vi "day 7 task 2.vi"() -> ()   [LabVIEW 2019]
panel:
  out "deleteme":u64
  out "sum pt 1":u64
  out "element":map{string, u64}(c390)
  out "String":string
  out "map":T1(c390)
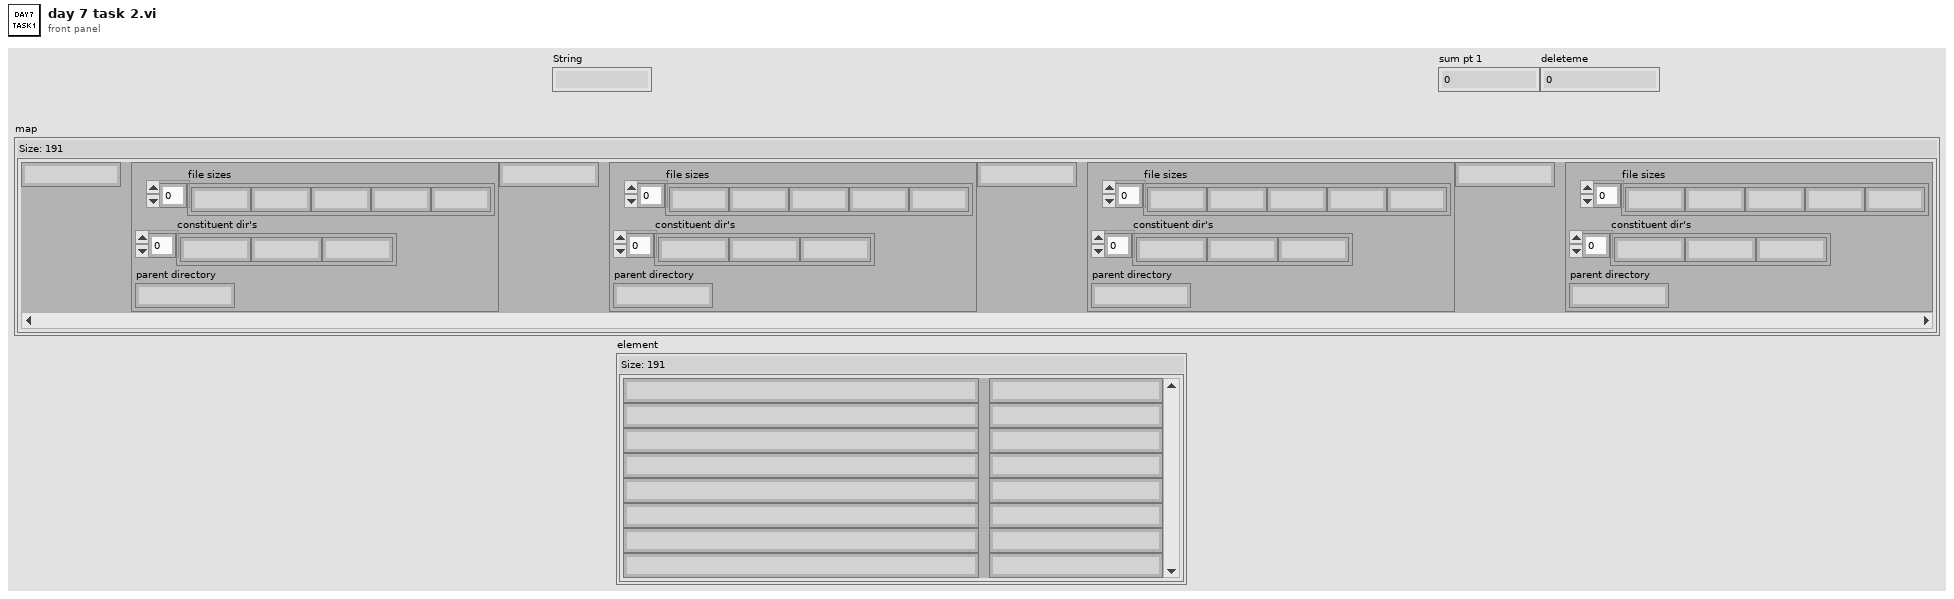
[diagram p1: front panel]
types:
  T1 = map{string, cluster{"file sizes":u64[], "constituent dir's":string[], "parent directory":string}}
  T2 = cluster{"file sizes":u64[], "constituent dir's":string[], "parent directory":string}
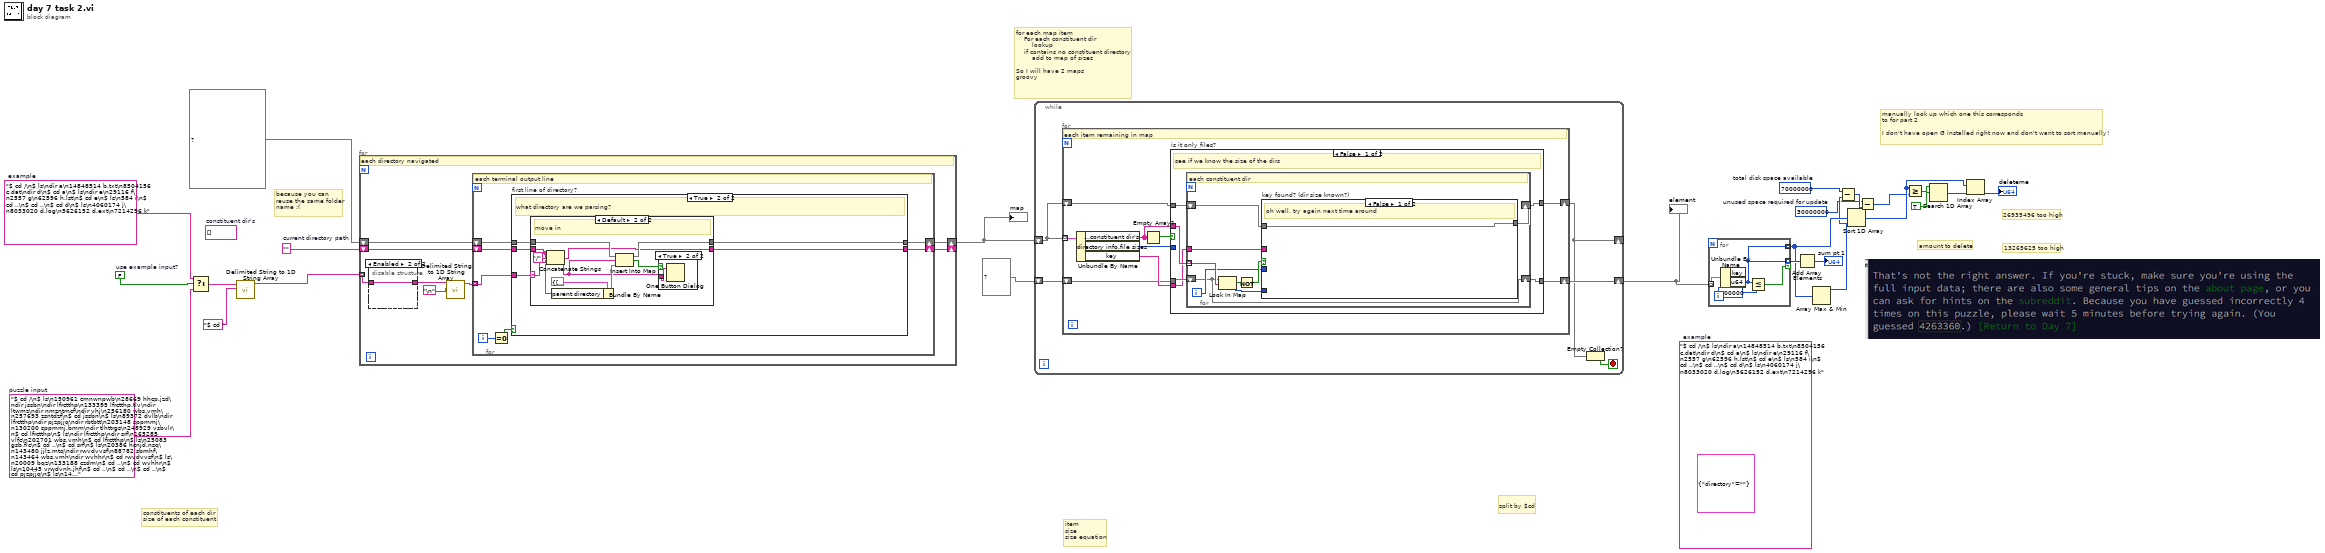
[diagram p0: block diagram]
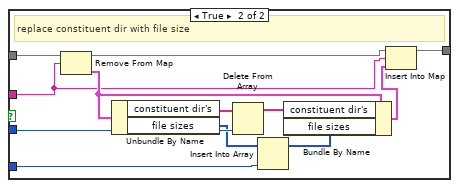
[diagram p2: hidden frame]
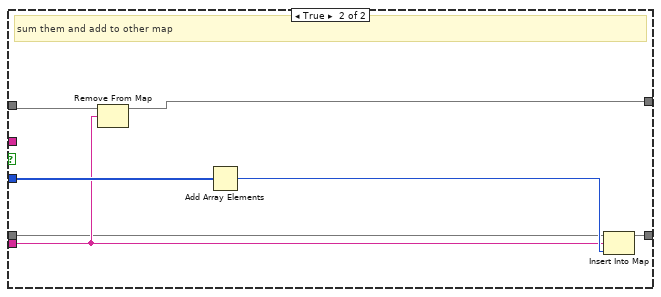
[diagram p3: hidden frame]
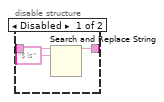
[diagram p4: hidden frame]
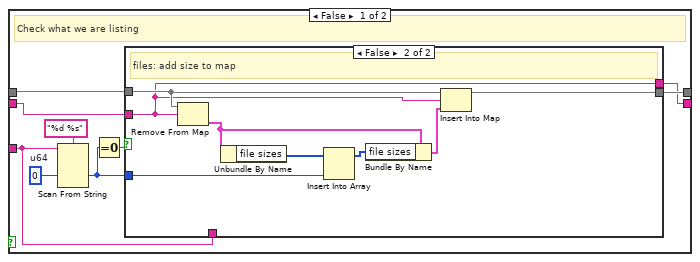
[diagram p5: hidden frame]
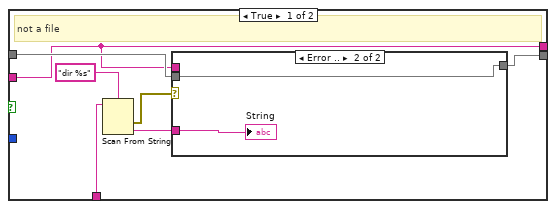
[diagram p6: hidden frame]
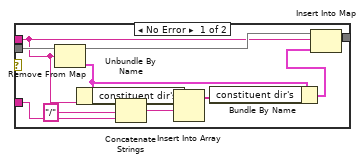
[diagram p7: hidden frame]
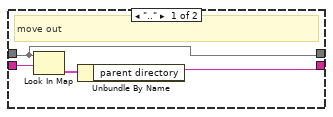
[diagram p8: hidden frame]
diagram:
  w1 = u64 30000000  # unused space required for update
  w12 = u64 70000000  # total disk space available
  w17 = ""  # current directory path
  (unwired) string[] []  # constituent dir's
  (unwired) cluster{"directory":string} {"directory"=""}
  (unwired) "$ cd /\n$ ls\ndir a\n14848514 b.txt\n8504156 c.dat\ndir d\n$ cd a\n$ ls\ndir e\n29116 f\n2557 g\n62596 h.lst\n$ cd e\n$ ls\n584 i\n$ cd ..\n$ cd ..\n$ cd d\n$ ls\n4060174 j\n8033020 d.log\n5626152 d.ext\n7214296 k"  # example
  w22 = "$ cd /\n$ ls\ndir a\n14848514 b.txt\n8504156 c.dat\ndir d\n$ cd a\n$ ls\ndir e\n29116 f\n2557 g\n62596 h.lst\n$ cd e\n$ ls\n584 i\n$ cd ..\n$ cd ..\n$ cd d\n$ ls\n4060174 j\n8033020 d.log\n5626152 d.ext\n7214296 k"  # example
  w23 = FALSE  # use example input?
  w24 = "$ cd /\n$ ls\n150961 cmnwnpwb\n28669 hhcp.jzd\ndir jssbn\ndir lfrctthp\n133395 lfrctthp.tlv\ndir ltwmz\ndir nmzntmcf\ndir vhj\n256180 wbs.vmh\n257693 zsntdzf\n$ cd jssbn\n$ ls\n89372 dvlb\ndir lfrctthp\ndir pjzpjjq\ndir rbtbtt\n203148 sppmmj\n130200 sppmmj.bmm\ndir tlhttrgs\n248929 vsbvlr\n$ cd lfrctthp\n$ ls\ndir lfrctthp\ndir srf\n165285 vlfc\n202701 wbs.vmh\n$ cd lfrctthp\n$ ls\n25083 gsb.flc\n$ cd ..\n$ cd srf\n$ ls\n20386 hcnjd.nsq\n143480 jjlz.mtq\ndir rwvdvvsf\n88782 sbmhf\n143464 wbs.vmh\ndir wvhhr\n$ cd rwvdvvsf\n$ ls\n20009 bqz\n133188 czdm\n$ cd ..\n$ cd wvhhr\n$ ls\n10445 vrwdvnh.jhf\n$ cd ..\n$ cd ..\n$ cd ..\n$ cd pjzpjjq\n$ ls\n14329 chgbd.zjf\ndir dvlb\n212284 pjc\ndir qlrn\n225566 rhzgmnb.nhd\n145766 sppmmj.dzz\ndir vpltwcs\n125853 wbs.vmh\n$ cd dvlb\n$ ls\ndir bjfqsb\ndir fnwsmj\n154127 gplzm\n264923 qcp.qvc\ndir wlhfvwl\ndir wrgqqts\ndir zhj\n$ cd bjfqsb\n$ ls\ndir jgltcw\n$ cd jgltcw\n$ ls\n264579 shmqqjf.fwd\n$ cd ..\n$ cd ..\n$ cd fnwsmj\n$ ls\ndir lfrctthp\ndir rddpmj\n$ cd lfrctthp\n$ ls\ndir qdgqdtn\n198919 qhjbh.fbc\ndir sgddcfdn\n$ cd qdgqdtn\n$ ls\n230357 lbcgfp.vzq\n$ cd ..\n$ cd sgddcfdn\n$ ls\n110212 cwjbzd.npb\ndir lnjln\n207550 wlvdsjj\n$ cd lnjln\n$ ls\n28970 tdw\n$ cd ..\n$ cd ..\n$ cd ..\n$ cd rddpmj\n$ ls\ndir fhlnmw\n$ cd fhlnmw\n$ ls\n228871 mcgdrzg\n$ cd ..\n$ cd ..\n$ cd ..\n$ cd wlhfvwl\n$ ls\ndir rbwq\n$ cd rbwq\n$ ls\n139444 jdczdlwb\n66039 mnbq.sdq\n$ cd ..\n$ cd ..\n$ cd wrgqqts\n$ ls\n124869 dvlb.cfl\n$ cd ..\n$ cd zhj\n$ ls\ndir hww\n192363 lqn\ndir nqv\n$ cd hww\n$ ls\n14681 czhd.bdn\n232222 fgcfbrs.wqt\ndir pnsbrd\n155416 vsw.npv\n199792 wbs.vmh\n44877 znpdrr.rmd\n$ cd pnsbrd\n$ ls\n179442 vsbvlr\n55431 zbhj.wnh\n$ cd ..\n$ cd ..\n$ cd nqv\n$ ls\n262693 hnz.czd\n259429 lptljbz\ndir rjgbm\ndir tlhttrgs\n76496 tlhttrgs.jlv\n260003 vsbvlr\n$ cd rjgbm\n$ ls\n45885 fgfh.tch\n42899 lfrctthp.fbc\n159401 nnmg.tvz\n144595 trzgtn.scg\n$ cd ..\n$ cd tlhttrgs\n$ ls\ndir cqtnvzn\n220458 wbs.vmh\n$ cd cqtnvzn\n$ ls\n49609 czdm\n$ cd ..\n$ cd ..\n$ cd ..\n$ cd ..\n$ cd ..\n$ cd qlrn\n$ ls\n150270 bflnzt\n203988 bgq\ndir jwgd\n256702 sppmmj\ndir wbgvqpc\n$ cd jwgd\n$ ls\n57414 lmlbtpg.wdp\n$ cd ..\n$ cd wbgvqpc\n$ ls\ndir dvlb\ndir qfhvjtv\ndir tpcwhmv\n$ cd dvlb\n$ ls\n118388 hhcp.jzd\n$ cd ..\n$ cd qfhvjtv\n$ ls\n82966 lfrctthp\ndir mhbbpdpj\n139234 wbs.vmh\n$ cd mhbbpdpj\n$ ls\ndir ghrbbh\n$ cd ghrbbh\n$ ls\n24686 tlhttrgs\n$ cd ..\n$ cd ..\n$ cd ..\n$ cd tpcwhmv\n$ ls\n3666 hhcp.jzd\n$ cd ..\n$ cd ..\n$ cd ..\n$ cd vpltwcs\n$ ls\ndir tlhttrgs\n146745 vsbvlr\n$ cd tlhttrgs\n$ ls\ndir cchd\n32682 cvbr.rmh\n209102 mpdpnb\n96179 wbs.vmh\n$ cd cchd\n$ ls\n126044 wmrv\n$ cd ..\n$ cd ..\n$ cd ..\n$ cd ..\n$ cd rbtbtt\n$ ls\n169793 hzgdsb.tbs\ndir wqmvzg\n$ cd wqmvzg\n$ ls\ndir lzbj\n$ cd lzbj\n$ ls\ndir tnhdmqjh\n$ cd tnhdmqjh\n$ ls\n5150 lfrctthp\n$ cd ..\n$ cd ..\n$ cd ..\n$ cd ..\n$ cd tlhttrgs\n$ ls\ndir zjghthcb\ndir zmlpwlm\n$ cd zjghthcb\n$ ls\ndir dvlb\ndir ghzsqrn\ndir hvwjc\ndir lfrctthp\n$ cd dvlb\n$ ls\n167639 dvlb.fhs\n70305 qnhgn.mgn\n$ cd ..\n$ cd ghzsqrn\n$ ls\n74556 dbrtz.lrn\ndir fngzpjm\ndir mdqbvhrr\n220711 mrfjpgwj\ndir sfhqmzhd\n67424 tlhttrgs.thf\n202325 vsngvn.ttq\n$ cd fngzpjm\n$ ls\ndir dvlb\ndir ghzwdw\n$ cd dvlb\n$ ls\n59824 bmvzg\n184952 lfrctthp\n51434 qwcttnh.pbs\n206348 wbs.vmh\n$ cd ..\n$ cd ghzwdw\n$ ls\n132594 lfrctthp\n99032 tlhttrgs.cvp\n$ cd ..\n$ cd ..\n$ cd mdqbvhrr\n$ ls\n32598 zsfv.qqv\n$ cd ..\n$ cd sfhqmzhd\n$ ls\n58893 wpmbm\n$ cd ..\n$ cd ..\n$ cd hvwjc\n$ ls\n233454 ccpnsjm.cwc\n72232 lfrctthp\ndir nchvqtdq\n248368 ptrlpt.gdf\n222059 qgjv\n69105 wbs.vmh\ndir wnj\n$ cd nchvqtdq\n$ ls\n49931 gjwjq.jrc\n$ cd ..\n$ cd wnj\n$ ls\n182139 ccpnsjm.cwc\ndir dvlb\n72806 hhcp.jzd\n156378 sppmmj\n$ cd dvlb\n$ ls\ndir cwjbzd\n$ cd cwjbzd\n$ ls\ndir tlhttrgs\n$ cd tlhttrgs\n$ ls\n240264 vdp.wzt\n$ cd ..\n$ cd ..\n$ cd ..\n$ cd ..\n$ cd ..\n$ cd lfrctthp\n$ ls\n168164 ccpnsjm.cwc\n68428 dcmfjn\n133121 dvlb\n146217 sppmmj.zjm\ndir thgh\ndir zzffz\n$ cd thgh\n$ ls\ndir nrntbh\ndir qlhbf\n$ cd nrntbh\n$ ls\n139964 lfrctthp.brp\n$ cd ..\n$ cd qlhbf\n$ ls\n115891 vsbvlr\n$ cd ..\n$ cd ..\n$ cd zzffz\n$ ls\n170513 tlhttrgs.hsw\n$ cd ..\n$ cd ..\n$ cd ..\n$ cd zmlpwlm\n$ ls\n232644 wvjrtvps.hrb\n$ cd ..\n$ cd ..\n$ cd ..\n$ cd lfrctthp\n$ ls\ndir cwjbzd\ndir dvlb\n65658 fclf\n191985 hhcp.jzd\ndir lwqdqm\ndir mpb\ndir ndn\ndir rtpwjds\n185299 smp\ndir sqhvvsb\ndir vzh\ndir zzvnq\n$ cd cwjbzd\n$ ls\n172122 ccpnsjm.cwc\ndir dfqpqqw\ndir lfrctthp\n123102 lfrctthp.cms\n73991 lqhjcbms\n207693 mcnwp\ndir sppmmj\n114128 tzrrgl\n$ cd dfqpqqw\n$ ls\n67239 dgssm.crl\ndir rjm\n$ cd rjm\n$ ls\n25830 nnwdzf\n$ cd ..\n$ cd ..\n$ cd lfrctthp\n$ ls\ndir fqswn\n241343 jllwj.wjc\n$ cd fqswn\n$ ls\n76154 ccpnsjm.cwc\ndir dhgghnm\ndir vpbwj\n$ cd dhgghnm\n$ ls\n36757 jbmlssv.ndp\ndir sppmmj\n$ cd sppmmj\n$ ls\ndir dsss\n$ cd dsss\n$ ls\n201519 vsbvlr\n$ cd ..\n$ cd ..\n$ cd ..\n$ cd vpbwj\n$ ls\n154042 ccpnsjm.cwc\ndir tlhttrgs\n271666 vsbvlr\n$ cd tlhttrgs\n$ ls\n125785 cwjbzd.lqr\n19315 jdcm.mrz\n$ cd ..\n$ cd ..\n$ cd ..\n$ cd ..\n$ cd sppmmj\n$ ls\ndir sppmmj\n$ cd sppmmj\n$ ls\n161387 fwh.wtt\n$ cd ..\n$ cd ..\n$ cd ..\n$ cd dvlb\n$ ls\ndir dnqvhtr\ndir jqpzj\ndir jvvsgbl\ndir tlhttrgs\n$ cd dnqvhtr\n$ ls\ndir jzm\ndir phcfgqfs\ndir sppmmj\ndir vhrst\n$ cd jzm\n$ ls\n143413 sgsbj.qtr\ndir smtpdcpf\n$ cd smtpdcpf\n$ ls\n95947 lgzlj\n$ cd ..\n$ cd ..\n$ cd phcfgqfs\n$ ls\n257801 hhcp.jzd\n$ cd ..\n$ cd sppmmj\n$ ls\n230280 ccpnsjm.cwc\n261954 hhcp.jzd\ndir hmcn\ndir mrhsrrm\ndir nlqmghj\ndir rqbtcvfw\n70788 vsbvlr\n114344 wbs.vmh\n225265 wjnf.wrv\n$ cd hmcn\n$ ls\n206476 dvlb\n214973 lfrctthp\n$ cd ..\n$ cd mrhsrrm\n$ ls\n126589 wbs.vmh\n$ cd ..\n$ cd nlqmghj\n$ ls\n113621 mdqvh.flp\n$ cd ..\n$ cd rqbtcvfw\n$ ls\n259673 wbs.vmh\n$ cd ..\n$ cd ..\n$ cd vhrst\n$ ls\n102273 sppmmj\n$ cd ..\n$ cd ..\n$ cd jqpzj\n$ ls\n7675 vwls.wjz\n$ cd ..\n$ cd jvvsgbl\n$ ls\n217539 bgjgtfbv.wcf\ndir fbvls\ndir gtwrhhd\ndir tlhttrgs\n59720 wbs.vmh\n$ cd fbvls\n$ ls\n146823 ccpnsjm.cwc\n$ cd ..\n$ cd gtwrhhd\n$ ls\n59762 wbs.vmh\n$ cd ..\n$ cd tlhttrgs\n$ ls\n7093 ccpnsjm.cwc\ndir dvlb\ndir hjclnb\n$ cd dvlb\n$ ls\n62683 trww\n$ cd ..\n$ cd hjclnb\n$ ls\n245444 bcnlmstj.bsj\n167166 czdm\n$ cd ..\n$ cd ..\n$ cd ..\n$ cd tlhttrgs\n$ ls\n53060 czdm\n217177 hzwn\n$ cd ..\n$ cd ..\n$ cd lwqdqm\n$ ls\ndir bdgnmf\ndir dvlb\n89596 vsbvlr\n$ cd bdgnmf\n$ ls\n146880 wbs.vmh\n$ cd ..\n$ cd dvlb\n$ ls\n184438 vsbvlr\n$ cd ..\n$ cd ..\n$ cd mpb\n$ ls\ndir dvlb\n$ cd dvlb\n$ ls\ndir prqfqf\n$ cd prqfqf\n$ ls\ndir ltmjppj\n$ cd ltmjppj\n$ ls\n241963 bjgzsq.srr\n$ cd ..\n$ cd ..\n$ cd ..\n$ cd ..\n$ cd ndn\n$ ls\n184702 cnv.vtn\n52486 dvlb\ndir hfq\n52100 hswnvlq.frd\n$ cd hfq\n$ ls\ndir bsjgglbs\n263904 cwjbzd.sht\n265639 phpvlfw.jmm\n178105 wbs.vmh\n25124 wcq.qct\n$ cd bsjgglbs\n$ ls\n121761 czdm\n$ cd ..\n$ cd ..\n$ cd ..\n$ cd rtpwjds\n$ ls\n117111 qjvrwsfl\n132235 rwjf\ndir sdssvrst\n223399 wjfdgt.ldj\n$ cd sdssvrst\n$ ls\n114380 ccpnsjm.cwc\n$ cd ..\n$ cd ..\n$ cd sqhvvsb\n$ ls\n7812 gjhj\n239114 hhcp.jzd\ndir ldmwm\n230777 vsbvlr\n$ cd ldmwm\n$ ls\n67855 blcbqb.wpz\ndir cwjbzd\n250365 czdm\n249613 dvlb.mfq\ndir jdsbt\n95934 tlhttrgs.wgw\n$ cd cwjbzd\n$ ls\n147822 cwjbzd.lff\n122632 hhcp.jzd\ndir llcflrds\ndir tlhttrgs\n67326 tvptb.fzl\ndir wtcttdzg\n$ cd llcflrds\n$ ls\ndir cngdgq\n$ cd cngdgq\n$ ls\n235724 lqqcfphg\n$ cd ..\n$ cd ..\n$ cd tlhttrgs\n$ ls\ndir cgf\n67714 csb.hcw\ndir cwjbzd\ndir jvs\n119180 lfrctthp.qgm\ndir ppsmqwn\ndir qqmtj\ndir qzmpwzvz\ndir zmsbqrqf\n$ cd cgf\n$ ls\ndir dvlb\n$ cd dvlb\n$ ls\n77864 thff\n$ cd ..\n$ cd ..\n$ cd cwjbzd\n$ ls\n208459 ccpnsjm.cwc\n17127 dtqglmf.zgb\n$ cd ..\n$ cd jvs\n$ ls\n142337 cwjbzd\n$ cd ..\n$ cd ppsmqwn\n$ ls\n147277 rmwh\n$ cd ..\n$ cd qqmtj\n$ ls\n153442 vqld.lsd\n$ cd ..\n$ cd qzmpwzvz\n$ ls\n223666 cwjbzd.gjl\n254370 gjc\n$ cd ..\n$ cd zmsbqrqf\n$ ls\n193665 tjwclf.nzs\n$ cd ..\n$ cd ..\n$ cd wtcttdzg\n$ ls\n52882 hhcp.jzd\n110104 hqwgl.mtb\n$ cd ..\n$ cd ..\n$ cd jdsbt\n$ ls\n77115 ccpnsjm.cwc\n242705 dvlb\n12624 lfrctthp\n145552 sppmmj\n198997 vsbvlr\n$ cd ..\n$ cd ..\n$ cd ..\n$ cd vzh\n$ ls\ndir ccbjg\n91733 czdm\n89195 dvlb\n212167 rvfpbl.rtq\n224909 tlhttrgs.djt\n72916 vpznzhs.dcd\n$ cd ccbjg\n$ ls\ndir mcvsbd\ndir sppmmj\n$ cd mcvsbd\n$ ls\ndir cwjbzd\ndir rbsv\n$ cd cwjbzd\n$ ls\n224826 ccpnsjm.cwc\n$ cd ..\n$ cd rbsv\n$ ls\n164816 lfrctthp\n$ cd ..\n$ cd ..\n$ cd sppmmj\n$ ls\n85264 ccpnsjm.cwc\n104511 dvlb.qgj\n183533 lfrctthp.zdn\n98525 wbs.vmh\n$ cd ..\n$ cd ..\n$ cd ..\n$ cd zzvnq\n$ ls\n107390 lfrctthp\ndir lznpqbrd\ndir pddfg\n143496 prnjh.sgb\ndir pvdz\ndir vnmhs\n118674 zhnh.mpl\n$ cd lznpqbrd\n$ ls\n157950 dpvcgj.wlw\ndir dvlb\n175412 dvlb.qvr\ndir lfrctthp\n84587 pmsjdj\n$ cd dvlb\n$ ls\n41223 rwr.nbz\n$ cd ..\n$ cd lfrctthp\n$ ls\n26056 fqc.fnl\n28191 lgjlw.vql\ndir sppmmj\n262066 wbs.vmh\n$ cd sppmmj\n$ ls\n246742 ccpnsjm.cwc\n$ cd ..\n$ cd ..\n$ cd ..\n$ cd pddfg\n$ ls\ndir cwjbzd\ndir jbw\n147410 vsbvlr\n$ cd cwjbzd\n$ ls\n197956 jpzb.dcw\n$ cd ..\n$ cd jbw\n$ ls\n247206 vsbvlr\n$ cd ..\n$ cd ..\n$ cd pvdz\n$ ls\ndir jctpqbgw\n153177 qwcgjttm.lzm\n94686 vsbvlr\n$ cd jctpqbgw\n$ ls\n190424 qvm\n$ cd ..\n$ cd ..\n$ cd vnmhs\n$ ls\n16118 sdhmzhlg.blf\n$ cd ..\n$ cd ..\n$ cd ..\n$ cd ltwmz\n$ ls\n243152 bdmz\n$ cd ..\n$ cd nmzntmcf\n$ ls\ndir jqcms\ndir lrtsts\ndir lvchpdf\ndir qpzqp\ndir qrgh\ndir scwnmrds\n$ cd jqcms\n$ ls\n105562 ccpnsjm.cwc\n257512 chpr.zvl\ndir cwjbzd\ndir jzqbnpn\ndir ssr\n117496 tlhttrgs.thg\n72550 vsbvlr\n$ cd cwjbzd\n$ ls\ndir mwvlhzdn\ndir qrpllg\n205638 sppmmj.gcz\n$ cd mwvlhzdn\n$ ls\n272658 dvlb.bbw\n$ cd ..\n$ cd qrpllg\n$ ls\n215810 wbs.vmh\n$ cd ..\n$ cd ..\n$ cd jzqbnpn\n$ ls\n112583 sppmmj\n$ cd ..\n$ cd ssr\n$ ls\n66781 hpfpw.pvn\n138840 zhwplzd.wrq\n$ cd ..\n$ cd ..\n$ cd lrtsts\n$ ls\ndir drtrdnsg\n41195 dvlb.fgt\ndir lfrctthp\n$ cd drtrdnsg\n$ ls\ndir gnc\ndir sppmmj\n$ cd gnc\n$ ls\n127922 ccpnsjm.cwc\n233097 lfrctthp\n24075 qtglzq\n$ cd ..\n$ cd sppmmj\n$ ls\n128955 czdm\n64809 jtjh.nzq\ndir mdmh\ndir nbzh\n126095 wbs.vmh\ndir wwhbgg\n$ cd mdmh\n$ ls\ndir zvtjfz\n$ cd zvtjfz\n$ ls\n142470 ptp.qbf\n$ cd ..\n$ cd ..\n$ cd nbzh\n$ ls\n7112 ccpnsjm.cwc\n215395 chrtbjf.fwr\n145865 wld.pdl\n$ cd ..\n$ cd wwhbgg\n$ ls\n51752 hhcp.jzd\n$ cd ..\n$ cd ..\n$ cd ..\n$ cd lfrctthp\n$ ls\n198780 hhcp.jzd\n$ cd ..\n$ cd ..\n$ cd lvchpdf\n$ ls\n108580 hhcp.jzd\n105301 jpjjhshl\ndir njfmmj\ndir nsw\ndir sppmmj\ndir tlhttrgs\ndir tvsvr\n$ cd njfmmj\n$ ls\ndir bjsvdfrf\ndir gjgftj\ndir sppmmj\n25879 twzprtcf.hgl\n$ cd bjsvdfrf\n$ ls\n77668 vsbvlr\n$ cd ..\n$ cd gjgftj\n$ ls\ndir mjbw\n56593 vsbvlr\n$ cd mjbw\n$ ls\n243595 ccpnsjm.cwc\n$ cd ..\n$ cd ..\n$ cd sppmmj\n$ ls\ndir qzvwhr\n$ cd qzvwhr\n$ ls\ndir cwjbzd\n$ cd cwjbzd\n$ ls\n262825 wbs.vmh\n$ cd ..\n$ cd ..\n$ cd ..\n$ cd ..\n$ cd nsw\n$ ls\n210254 rgqpq\n$ cd ..\n$ cd sppmmj\n$ ls\n55463 cwjbzd.dtt\n196779 dvlb\n125377 hgb.qmj\ndir rdd\ndir tlhttrgs\n222280 tspz\ndir zbq\n$ cd rdd\n$ ls\n20045 srmsmr\n$ cd ..\n$ cd tlhttrgs\n$ ls\n47256 wbs.vmh\n$ cd ..\n$ cd zbq\n$ ls\n223951 cwjbzd.vrm\n$ cd ..\n$ cd ..\n$ cd tlhttrgs\n$ ls\n56808 jvndrcmd.ftl\ndir mjcmhg\n220385 prh.wtz\n231575 pzbtlg.fzv\n11100 sqfr.lzs\ndir tlhttrgs\n$ cd mjcmhg\n$ ls\n214188 llsfnv.dmc\n$ cd ..\n$ cd tlhttrgs\n$ ls\ndir qtws\ndir sbhswjld\n$ cd qtws\n$ ls\n102462 vjlwzbsg.whn\n$ cd ..\n$ cd sbhswjld\n$ ls\n159193 dvlb.bqj\n17424 hhcp.jzd\n28945 pdwrmgs.lzq\n38201 rpbllgs.rzn\ndir sppmmj\n$ cd sppmmj\n$ ls\n88100 wbs.vmh\n$ cd ..\n$ cd ..\n$ cd ..\n$ cd ..\n$ cd tvsvr\n$ ls\n237626 tlhttrgs.mhw\n$ cd ..\n$ cd ..\n$ cd qpzqp\n$ ls\ndir ddclns\n134373 lfrctthp\n167788 lstwpqbq.wln\n224743 qcplm\n14385 vzjj.bzm\n108204 wbs.vmh\n$ cd ddclns\n$ ls\ndir vprlq\n$ cd vprlq\n$ ls\n137784 ccpnsjm.cwc\n$ cd ..\n$ cd ..\n$ cd ..\n$ cd qrgh\n$ ls\n29875 ccpnsjm.cwc\n225323 hhcp.jzd\n135470 tlhttrgs\n23724 vsbvlr\n$ cd ..\n$ cd scwnmrds\n$ ls\ndir sppmmj\n$ cd sppmmj\n$ ls\ndir sppmmj\n$ cd sppmmj\n$ ls\n73173 blznf.smd\n$ cd ..\n$ cd ..\n$ cd ..\n$ cd ..\n$ cd vhj\n$ ls\n221377 cwjbzd.tvv\n98748 czdm\n108605 hhcp.jzd\ndir jnm\ndir lfrctthp\n11518 lfrctthp.jfl\n89038 psnfcwpq.zcd\ndir tlhttrgs\n$ cd jnm\n$ ls\n66785 bfwm\n196636 dssh.rwn\ndir sppmmj\n140177 tlhttrgs.jlh\n199730 vsbvlr\n$ cd sppmmj\n$ ls\n101586 ccpnsjm.cwc\ndir lfrctthp\n127582 vsbvlr\n71001 zvrzs\n$ cd lfrctthp\n$ ls\n122902 lfrctthp\n247157 svmpmrl.tcc\n$ cd ..\n$ cd ..\n$ cd ..\n$ cd lfrctthp\n$ ls\n104555 cwjbzd.hbf\n56298 pldmc.hjd\n27639 sppmmj.nmr\n$ cd ..\n$ cd tlhttrgs\n$ ls\n252680 zsjgqqb"  # puzzle input
  # "13265625 too high"
  # "26935496 too high"
  # "manually look up which one this corresponds\nto for part 2\n\nI don't have open G installed right now and don't want to sort manually!"
  # "amount to delete"
  # "because you can \nreuse the same folder\nname :("
  # "for each map item\n    For each constituent dir\n        lookup\n    if contains no constituent directory\n        add to map of sizes\n\nSo I will have 2 maps\ngroovy"
  # "split by $cd"
  # "item\nsize\nsize equation"
  # "constituents of each dir\nsize of each constituent"
  n1 = Select(t=w22, s=w23, f=w24) -> (s? t:f=w21:string)
  n2 = call <vilib>:"Delimited String to 1D String Array.vi"("delimiter"="$ cd ", "delimited string"=w21) -> ("string array"=w19:string[])  [unwired: 9 in]
  n3 = for {
    tunnel: w19 -> [w29] mode=indexing
    shift-right: [w27] -> _
    shift-left: w17 -> [w26]
    shift-right: [w25] -> w16
    shift-left: T1 {} ("map") -> [w28]
    # "each directory navigated"
    n4 = disable-structure shown="Enabled" {
      disable-tunnel: [w35 w36] -> w30
      disable-tunnel: w29 -> [w34 w36]
      frame Disabled {
        n5 = Search and Replace String(input string=w34, search string="$ ls") -> (result string=w35:string)  [unwired: 6 in, 3 out]
      }
      frame Enabled {
      }
    }
    n6 = call <vilib>:"Delimited String to 1D String Array.vi"("delimiter"="\n", "delimited string"=w30) -> ("string array"=w31:string[])  [unwired: 9 in]
    n7 = for {
      tunnel: w31 -> [w42] mode=indexing
      shift-right: [w39] -> w27
      shift-left: w26 -> [w38]
      shift-right: [w37] -> w25
      shift-left: w28 -> [w40]
      i -> [w43]
      # "each terminal output line"
      n8 = Equal To 0?(x=w43) -> (x = 0?=w41:bool)
      n9 = case "first line of directory?" shown="True" w41 {
        tunnel: w42 -> [w47 w85]
        tunnel: w40 -> [w49 w84]
        tunnel: [w46 w83] -> w39
        tunnel: w38 -> [w48 w82]
        tunnel: [w50 w81] -> w37
        frame False {
          w52 = u64 0  # u64
          # "Check what we are listing"
          n10 = Scan From String(format string="%d %s", input string=w47, default 1=w52) -> (output 1=w45:u64)  [unwired: 4 in, 3 out]
          n11 = Equal To 0?(x=w45) -> (x = 0?=w44:bool)
          n12 = case "file?" shown="False" w44 {
            tunnel: [w55 w80] -> w50
            tunnel: w49 -> [w56 w79]
            tunnel: w45 -> [_ w77]
            tunnel: w48 -> [w54 w73]
            tunnel: w47 -> [w58 _]
            tunnel: [w54 w73] -> w46
            frame True {
              # "not a file"
              n13 = Scan From String(format string="dir %s", input string=w58) -> (error out=w57:errorcluster, output 1=w53:string)  [unwired: 3 in, 2 out]
              n14 = case shown="Error .." w57 {
                tunnel: w56 -> [w67 w72]
                tunnel: [w65 w72] -> w55
                tunnel: w54 -> [w61 _]
                tunnel: w53 -> [w62 w71]
                frame No Error {
                  n15 = Remove From Map(10:w61, 11:w67) -> (1:w69:T2, 3:w66:T1)  [unwired: 1 out]
                  n16 = Unbundle By Name(w69) -> ("constituent dir's"=w70:string[])
                  n17 = Concatenate Strings(w61, "/" ("string"), w62) -> (w63:string)
                  n18 = Insert Into Array(array=w70, new element=w63) -> (w68:string[])  [unwired: 1 in]
                  n19 = Bundle By Name(cluster=w69, "constituent dir's"=w68) -> (w64:T2)
                  n20 = Insert Into Map(map in=w66, key=w61, value=w64) -> (map out=w65:T1)  [unwired: 2 out]
                }
                frame Error {
                  "String" <- w71
                }
              }
            }
            frame False {
              # "files: add size to map"
              n21 = Remove From Map(10:w73, 11:w79) -> (1:w76:T2)  [unwired: 2 out]
              n22 = Unbundle By Name(w76) -> ("file sizes"=w78:u64[])
              n23 = Insert Into Array(array=w78, new element=w77) -> (w75:u64[])  [unwired: 1 in]
              n24 = Bundle By Name(cluster=w76, "file sizes"=w75) -> (w74:T2)
              n25 = Insert Into Map(map in=w79, key=w73, value=w74) -> (map out=w80:T1)  [unwired: 2 out]
            }
          }
        }
        frame True {
          # "what directory are we parsing?"
          n26 = case shown="Default" w85 {
            selector: w85 -> [_ w92]
            tunnel: w84 -> [w86 w97]
            tunnel: [w87 w93] -> w83
            tunnel: w82 -> [w89 w90]
            tunnel: [w86 w98] -> w81
            frame ".." {
              # "move out"
              n27 = Look In Map(map=w86, key=w89) -> (value=w88:T2)  [unwired: 1 in, 1 out]
              n28 = Unbundle By Name(w88) -> ("parent directory"=w87:string)
            }
            frame Default {
              # "move in"
              n29 = Concatenate Strings(w90, "/" ("string"), w92) -> (w93:string)
              n30 = Bundle By Name(cluster=T2 {"file sizes"=[], "constituent dir's"=[], "parent directory"=""} ("value"), "parent directory"=w90) -> (w95:T2)
              n31 = Insert Into Map(map in=w97, key=w93, value=w95) -> (map out=w98:T1, key already included?=w94:bool)  [unwired: 1 out]
              n32 = case shown="True" w94 {
                tunnel: w93 -> [_ w99]
                frame False {
                }
                frame True {
                  n33 = One Button Dialog(message=w99) -> ()  [unwired: 1 in, 1 out]
                }
              }
            }
          }
        }
      }
    }
  }
  "map" <- w16
  n34 = while {
    shift-right: [w101] -> _
    shift-left: w16 -> [w102]
    shift-right: [w104] -> w14
    shift-left: map{string, u64} {} ("element") -> [w103]
    stop <- w100 stop-if-true
    n35 = for {
      tunnel: w102 -> [w110] mode=indexing
      shift-right: [w106] -> w101
      shift-left: w102 -> [w107]
      shift-right: [w105] -> w104
      shift-left: w103 -> [w111]
      # "each item remaining in map"
      n36 = Unbundle By Name(w110) -> ("directory info.constituent dir's"=w108:string[], "directory info.file sizes"=w113:u64[], "key"=w112:string)
      n37 = Empty Array?(array=w108) -> (empty?=w109:bool)
      n38 = case "is it only files?" shown="False" w109 {
        tunnel: w113 -> [_ w148]
        tunnel: w112 -> [w114 w145]
        tunnel: w111 -> [w116 w142]
        tunnel: w108 -> [w119 _]
        tunnel: w107 -> [w118 w146]
        tunnel: [w117 w144] -> w106
        tunnel: [w115 w143] -> w105
        frame False {
          # "see if we know the size of the dirs"
          n39 = for {
            tunnel: w119 -> [w127] mode=indexing
            shift-right: [w123] -> w117
            shift-left: w118 -> [w128]
            shift-right: [w122] -> w115
            shift-left: w116 -> [w122]
            tunnel: w114 -> [w120]
            i -> [w124]
            # "each constituent dir"
            n40 = Look In Map(map=w122, key=w127) -> (key not found?=w126:bool, value=w121:u64)  [unwired: 1 in]
            n41 = Not(x=w126) -> (.not. x?=w125:bool)
            n42 = case "key found? (dir size known?)" shown="False" w125 {
              tunnel: w128 -> [w129 w141]
              tunnel: w120 -> [_ w131]
              tunnel: w124 -> [_ w139]
              tunnel: [w129 w132] -> w123
              tunnel: w121 -> [_ w130]
              frame False {
                # "oh well, try again next time around"
              }
              frame True {
                # "replace constituent dir with file size"
                n43 = Remove From Map(10:w131, 11:w141) -> (1:w138:T2, 3:w137:T1)  [unwired: 1 out]
                n44 = Unbundle By Name(w138) -> ("constituent dir's"=w140:string[], "file sizes"=w134:u64[])
                n45 = Delete From Array(array=w140, index=w139) -> (array with subset deleted=w135:string[])  [unwired: 1 in, 1 out]
                n46 = Insert Into Array(array=w134, new element=w130) -> (w133:u64[])  [unwired: 1 in]
                n47 = Bundle By Name(cluster=w138, "constituent dir's"=w135, "file sizes"=w133) -> (w136:T2)
                n48 = Insert Into Map(map in=w137, key=w131, value=w136) -> (map out=w132:T1)  [unwired: 2 out]
              }
            }
          }
        }
        frame True {
          # "sum them and add to other map"
          n49 = Remove From Map(10:w145, 11:w146) -> (3:w144:T1)  [unwired: 2 out]
          n50 = Add Array Elements(numeric array=w148) -> (sum=w147:u64)
          n51 = Insert Into Map(map in=w142, key=w145, value=w147) -> (map out=w143:map{string, u64})  [unwired: 2 out]
        }
      }
    }
    n52 = Empty Collection?(1:w101) -> (0:w100:bool)
  }
  "element" <- w14
  n53 = for {
    tunnel: w14 -> [w152] mode=indexing
    tunnel: [w149] -> w6 mode=indexing if=w150
    tunnel: [w149] -> w4 mode=indexing
    n54 = Unbundle By Name(w152) -> ("u64"=w149:u64)  [unwired: 1 out]
    n55 = Less Or Equal?(x=w149, y=u64 100000) -> (x <= y?=w150:bool)
  }
  n56 = Add Array Elements(numeric array=w6) -> (sum=→"sum pt 1":u64)
  n57 = Array Max & Min(array=w4) -> (max value=w3:u64)  [unwired: 3 out]
  n58 = Subtract(x=w12, y=w3) -> (x-y=w2:u64)
  n59 = Sort 1D Array(array=w4) -> (sorted array=w8:u64[])
  n60 = Subtract(x=w1, y=w2) -> (x-y=w5:u64)
  n61 = Greater Or Equal?(x=w8, y=w5) -> (x >= y?=w10:bool[])
  n62 = Search 1D Array(1D array=w10, element=TRUE) -> (index of element=w9:i32)  [unwired: 1 in]
  n63 = Index Array(array=w8, index=w9) -> (element=→"deleteme":u64)
